vi "Read Motor Angle Sensor 1.vi"(6 "error in":errorcluster, 8 "MaxRead":i32, 9 "Channel in":u16) -> (0 "error out":errorcluster, 1 "Messages":T1(array[cluster]), 2 "Pass":bool, 3 "Channel out":u16, 4 "Angle":dbl)   [LabVIEW 2023]
uses:
  7ad73885-74d4-4865-958d-ac69876d8a76.vi
  Communication/PCAN2023/PCAN API.lvlib
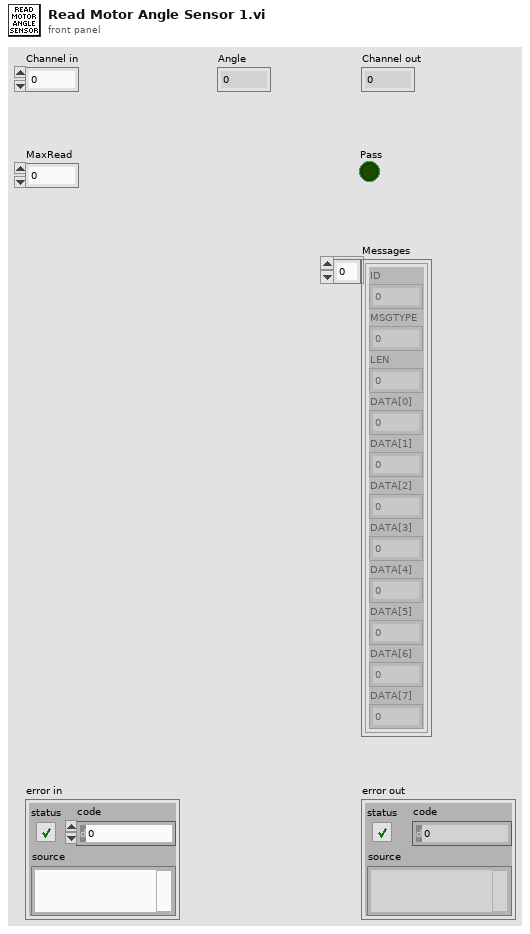
[diagram p1: front panel]
types:
  T1 = cluster{"ID":u32, "MSGTYPE":u8, "LEN":u8, "DATA[0]":u8, "DATA[1]":u8, "DATA[2]":u8, "DATA[3]":u8, "DATA[4]":u8, "DATA[5]":u8, "DATA[6]":u8, "DATA[7]":u8}[]
  T2 = cluster{"ID":u32, "MSGTYPE":u8, "LEN":u8, "DATA[0]":u8, "DATA[1]":u8, "DATA[2]":u8, "DATA[3]":u8, "DATA[4]":u8, "DATA[5]":u8, "DATA[6]":u8, "DATA[7]":u8}
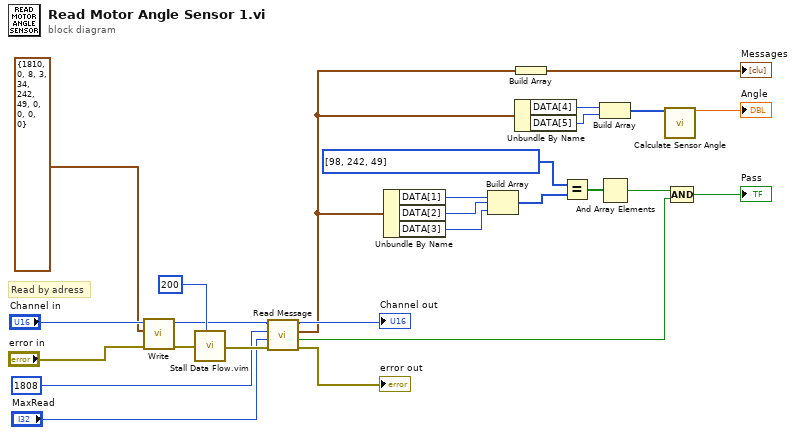
[diagram p0: block diagram]
diagram:
  # "Read by adress"
  n1 = call "Write.vi"("error in"="error in", "MessageBuffer"=T2 {"ID"=1810, "MSGTYPE"=0, "LEN"=8, "DATA[0]"=3, "DATA[1]"=34, "DATA[2]"=242, "DATA[3]"=49, "DATA[4]"=0, "DATA[5]"=0, "DATA[6]"=0, "DATA[7]"=0}, "Channel"="Channel in") -> ("error out"=w25:errorcluster, "Channel out"=w8:u16)  [unwired: 5 in, 2 out]
  n2 = call "Stall Data Flow.vim"("value in"=w25, "milliseconds to wait"=u32 200) -> ("value out"=w6:errorcluster)  [unwired: 1 out]
  n3 = call "Read Message.vi"("error in"=w6, "MaxRead"="MaxRead", "ID"=u32 1808, "Channel in"=w8) -> ("error out"=→"error out":errorcluster, "Passed"=w1:bool, "Last Message"=w2:T2, "Channel out"=→"Channel out":u16)  [unwired: 3 in, 1 out]
  n4 = Unbundle By Name(w2) -> ("DATA[1]"=w17:u8, "DATA[2]"=w15:u8, "DATA[3]"=w14:u8)
  n5 = Build Array(w17, w15, w14) -> (w16:u8[])
  n6 = Unbundle By Name(w2) -> ("DATA[4]"=w12:u8, "DATA[5]"=w11:u8)
  n7 = Build Array(w2) -> (→"Messages":T1)
  n8 = Equal?(x=u8[] [98, 242, 49], y=w16) -> (x = y?=w19:bool[])
  n9 = Build Array(w12, w11) -> (w10:u8[])
  n10 = And Array Elements(Boolean array=w19) -> (logical AND=w18:bool)
  n11 = call "Calculate Sensor Angle.vi"("DATA[4-5]"=w10) -> ("Degree0"=→"Angle":dbl)  [unwired: 17 in, 1 out]
  n12 = Compound Arithmetic op=AND(w18, w1) -> (→"Pass":bool)
